vi "Data_Save.vi"(6 "转置?":bool, 7 "path":path=path "D:/Save Data" caption="路径", 8 "Save_Data":string[](array[string]), 9 "Header":string[](array[string]), 10 "Save_Form":enum16{".txt", ".dat", ".xls", ".csv"}(ring), 11 "Save_Name":string) -> ()   [LabVIEW 2014]
uses:
  <vilib>/Utility/file.llb/Write To Spreadsheet File (string).vi
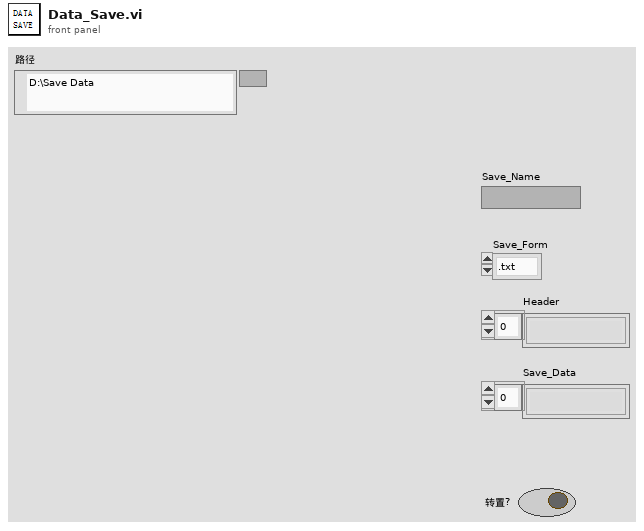
[diagram p1: front panel]
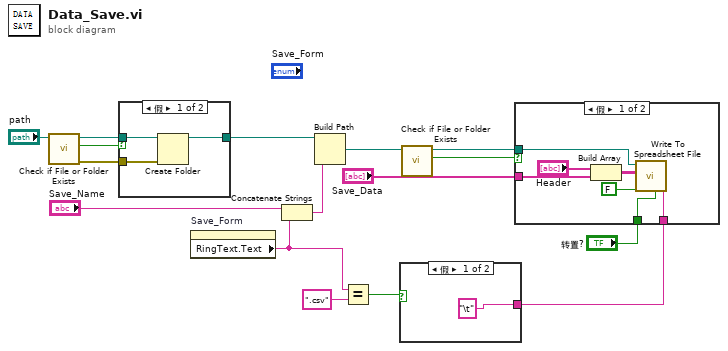
[diagram p0: block diagram]
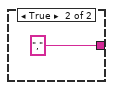
[diagram p2: hidden frame]
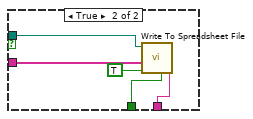
[diagram p3: hidden frame]
diagram:
  n1 = call <vilib>:"Check if File or Folder Exists.vi"("path"="path") -> ("error out"=w14:errorcluster, "file or folder exists?"=w16:bool, "dup path"=w15:path)  [unwired: 8 in]
  n2 = case shown="假" w16 {
    tunnel: w15 -> [w19 w20]
    tunnel: w14 -> [w18 _]
    tunnel: [w17 w20] -> w13
    frame False {
      n3 = Create Folder(path (use dialog)=w19, error in=w18) -> (created path=w17:path)  [unwired: 1 in, 2 out]
    }
    frame True {
    }
  }
  n4 = property on="Save_Form" class="Enum (严格)"() -> ("RingText.Text"=w5:string)  [unwired: 2 in, 2 out]
  n5 = Concatenate Strings("Save_Name", w5) -> (w12:string)
  n6 = Build Path(base path=w13, name or relative path=w12) -> (appended path=w10:path)
  n7 = Equal?(x=w5, y=".csv") -> (x = y?=w1:bool)
  n8 = case shown="假" w1 {
    tunnel: ["\t" ("delimiter (\\t)") "," ("delimiter (\\t)")] -> w3
    frame False {
    }
    frame True {
    }
  }
  n9 = call <vilib>:"Check if File or Folder Exists.vi"("path"=w10) -> ("file or folder exists?"=w9:bool, "dup path"=w7:path)  [unwired: 8 in, 1 out]
  n10 = case shown="假" w9 {
    tunnel: "Save_Data" -> [w28 w34]
    tunnel: w7 -> [w26 w32]
    tunnel: w3 -> [w24 w31]
    tunnel: "转置?" -> [w23 w30]
    frame False {
      n11 = Build Array("Header", w28) -> (w27:string[][])
      n12 = call-poly <vilib>:"Write To Spreadsheet File.vi"("delimiter (\\t)"=w24, "transpose? (no:F)"=w23, "append to file? (new file:F)"=FALSE, "2D data"=w27, "file path (dialog if empty)"=w26) -> ()  [unwired: 3 in, 1 out]
    }
    frame True {
      n13 = call-poly <vilib>:"Write To Spreadsheet File.vi"("delimiter (\\t)"=w31, "transpose? (no:F)"=w30, "append to file? (new file:F)"=TRUE, "1D data"=w34, "file path (dialog if empty)"=w32) -> ()  [unwired: 3 in, 1 out]
    }
  }
